vi "Set Position manually.vi"(8 "error in (no error)":errorcluster, 10 "Velocity value (units/s) in":dbl, 11 "Displacement (units)":dbl) -> (0 "error out":errorcluster, 3 "Current position (units)":dbl)   [LabVIEW 2011]
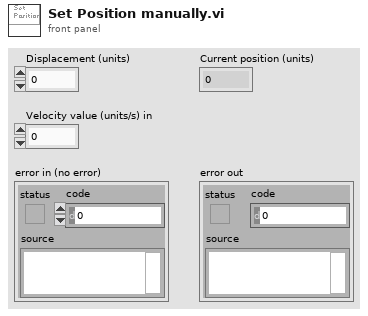
[diagram p1: front panel]
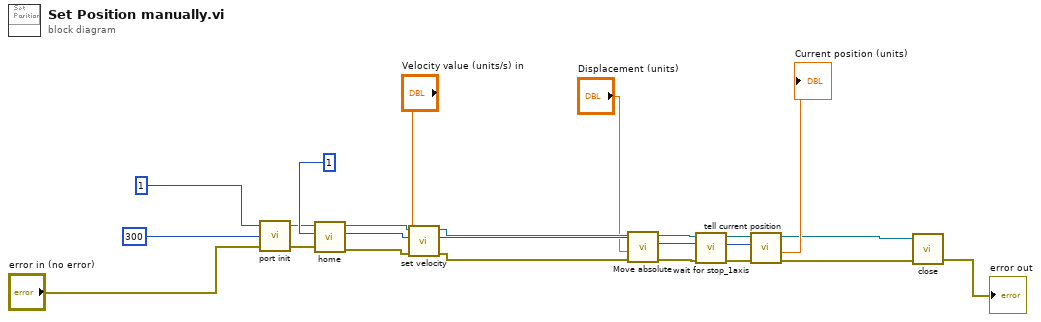
[diagram p0: block diagram]
diagram:
  n1 = call <userlib>:"port init.vi"("error in"="error in (no error)", "Timeout (ms)"=u32 300, "SerialPort"=u8 1) -> ("error out"=w8:errorcluster, "Visa Handle"=w7:refnum<visa-resource-name>)  [unwired: 1 in]
  n2 = call <userlib>:"home.vi"("error in"=w8, "Axis in"=1, "VISA Handle in"=w7) -> ("error out"=w17:errorcluster, "Axis out"=w16:i32, "VISA Handle out"=w15:refnum<visa-resource-name>)  [unwired: 3 in, 1 out]
  n3 = call <userlib>:"set velocity.vi"("error in"=w17, "Velocity value (units/s)"="Velocity value (units/s) in", "Axis in"=w16, "VISA Handle in"=w15) -> ("error out"=w20:errorcluster, "Axis out"=w21:i32, "VISA Handle out"=w19:refnum<visa-resource-name>)  [unwired: 2 in, 1 out]
  n4 = call <userlib>:"Move absolute.vi"("error in"=w20, "New target position (units)"="Displacement (units)", "Axis in"=w21, "VISA Handle in"=w19) -> ("error out"=w24:errorcluster, "Axis out"=w23:i32, "VISA Handle out"=w22:refnum<visa-resource-name>)  [unwired: 2 in, 1 out]
  n5 = call <userlib>:"wait for stop_1axis.vi"("error in"=w24, "Axis in"=w23, "VISA Handle in"=w22) -> ("error out"=w12:errorcluster, "Axis out"=w11:i32, "VISA Handle out"=w10:refnum<visa-resource-name>)  [unwired: 3 in, 1 out]
  n6 = call <userlib>:"tell current position.vi"("error in"=w12, "Axis in"=w11, "VISA Handle in"=w10) -> ("error out"=w1:errorcluster, "Current position (units)"=→"Current position (units)":dbl, "VISA Handle out"=w2:refnum<visa-resource-name>)  [unwired: 2 in, 2 out]
  n7 = call <userlib>:"close.vi"("error in"=w1, "VISA Handle in"=w2) -> ("error out"=→"error out":errorcluster)  [unwired: 3 in]
